vi "DereferencingPointerToArrayOfIntegersUsingMoveBlock.vi"(8 "error in (no error)":errorcluster, 10 "Length":i32, 11 "Address (Pointer)":i64) -> (0 "error out":errorcluster, 3 "Value":i32[](array[numeric]))   [LabVIEW 2009, in "LabVIEWWrapper_PassingDataSampleDLL.lvlib"]
uses:
  LabVIEWWrapper_PassingDataSampleDLL.lvlib
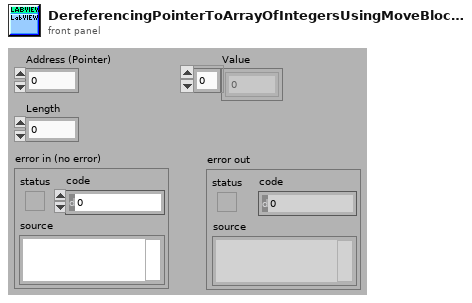
[diagram p1: front panel]
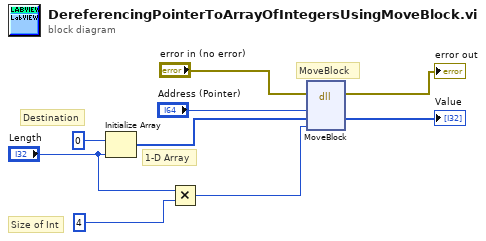
[diagram p0: block diagram]
diagram:
  # "1-D Array"
  # "Destination"
  # "Size of Int"
  # "MoveBlock"
  n1 = Initialize Array(0, "Length") -> (w5:i32[])
  n2 = Multiply(x="Length", y=4 ("arg3")) -> (x*y=w1:i32)
  n3 = dll-call lib="LabVIEW" fn="MoveBlock"(error in="error in (no error)", "Address (Pointer)"="Address (Pointer)", "Destination"=w5, "Size"=w1) -> (error out=→"error out":errorcluster, "Destination"=→"Value":i32[])  [unwired: 5 in, 1 out]
